vi "Get Member Relative Path.vi"(8 "error in (no error)":errorcluster, 10 "Member Name":string, 11 "LVLIBP Parser in":refnum<class "LVLIBP Parser.lvclass">) -> (0 "error out":errorcluster, 1 "Found ?":bool, 2 "Path":path, 3 "LVLIBP Parser out":refnum<class "LVLIBP Parser.lvclass">)   [LabVIEW 2018, in ".LVLIBP CD XML Updater.lvlib" / "LVLIBP Parser.lvclass"]
uses:
  LVLIBP Parser.lvclass
  LVLIBP Parser.lvclass/LVLIBP Parser.ctl
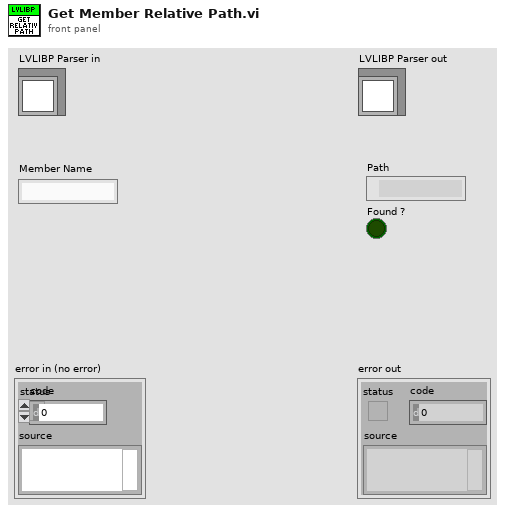
[diagram p1: front panel]
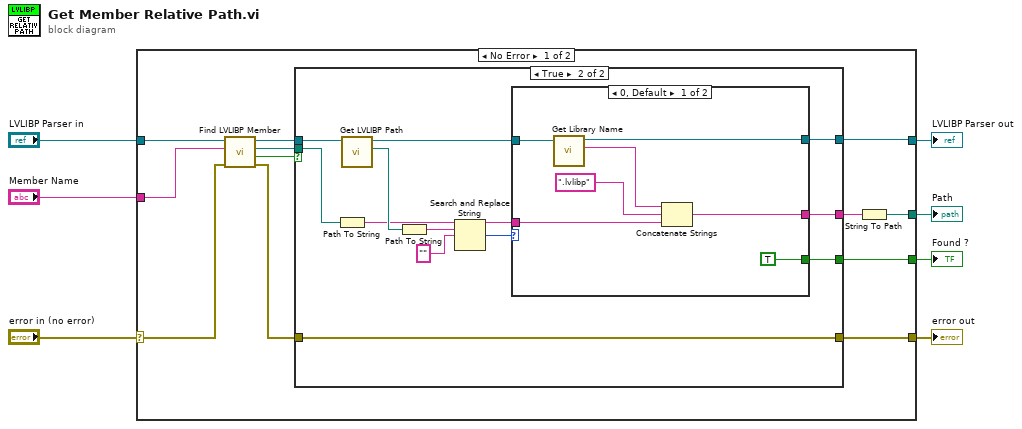
[diagram p0: block diagram]
diagram:
  n1 = case shown="No Error" "error in (no error)" {
    selector: "error in (no error)" -> [w10 w44]
    tunnel: [w8 w44] -> w6
    tunnel: [w14 w43] -> w4
    tunnel: "LVLIBP Parser in" -> [w19 w43]
    tunnel: "Member Name" -> [w18 _]
    tunnel: [w13 _] -> w2
    tunnel: [w11 _] -> w1
    frame No Error {
      n2 = call "Find LVLIBP Member.vi"("error in (no error)"=w10, "Member Name"=w18, "LVLIBP Parser in"=w19) -> ("error out"=w9:errorcluster, "Found ?"=w17:bool, "path"=w16:path, "LVLIBP Parser out"=w15:refnum<class "LVLIBP Parser.lvclass">)  [unwired: 5 in]
      n3 = case shown="True" w17 {
        tunnel: w16 -> [_ w32]
        tunnel: w15 -> [w21 w34]
        tunnel: [w21 w30] -> w14
        tunnel: [_ w29] -> w12
        tunnel: [_ w28] -> w13
        tunnel: w9 -> [w20 w27]
        tunnel: [w20 w27] -> w8
        frame False {
        }
        frame True {
          n4 = Path To String(path=w32) -> (string=w26:string)
          n5 = call "Get LVLIBP Path.vi"("LVLIBP Parser in"=w34) -> ("LVLIBP Path"=w33:path, "LVLIBP Parser out"=w31:refnum<class "LVLIBP Parser.lvclass">)  [unwired: 9 in]
          n6 = Path To String(path=w33) -> (string=w25:string)
          n7 = Search and Replace String(input string=w26, search string=w25, replace string="" ("replace string (\"\")")) -> (result string=w22:string, number of replacements=w24:i32)  [unwired: 5 in, 2 out]
          n8 = case shown="0, Default" w24 {
            tunnel: w31 -> [w41 w42]
            tunnel: [w38 w42] -> w30
            tunnel: [w37 _] -> w29
            tunnel: [TRUE _] -> w28
            tunnel: w22 -> [w35 _]
            frame 0, Default {
              n9 = call "Get Library Name.vi"("LVLIBP Parser in"=w41) -> ("Library Name"=w40:string, "LVLIBP Parser out"=w38:refnum<class "LVLIBP Parser.lvclass">)  [unwired: 9 in]
              n10 = Concatenate Strings(w40, ".lvlibp" ("string"), w35) -> (w37:string)
            }
            frame -1 {
            }
          }
        }
      }
      n11 = String To Path(string=w12) -> (path=w11:path)
    }
    frame Error {
    }
  }
  "error out" <- w6
  "LVLIBP Parser out" <- w4
  "Found ?" <- w2
  "Path" <- w1
